vi "increasing temp.vi"() -> ()   [LabVIEW 2016]
panel:
  in  "X":cluster{"Y":dbl[], "Y":dbl[]}[](graph)=[{"Y"=[3642203376.678899, 3642203381.4529734, 3642203385.471007, 3642203389.0781093, 3642203393.010663, 3642203396.7724032, 3642203404.0189867, 3642203408.627992, 3642203413.007674, 3642203417.017978, 3642203421.7605133, 3642203425.9109974, 3642203430.7061076, 3642203434.9230328, 3642203438.9979987, 3642203443.332184, 3642203447.2605352, 3642203451.7941136, 3642203459.39853, 3642203467.88641, 3642203474.175996, 3642203481.486995, 3642203488.474578, 3642203496.3469887, 3642203503.9469843, 3642203511.239989, 3642203517.483984, 3642203524.005077, 3642203531.319994, 3642203537.588065, 3642203544.0179725, 3642203549.2159953, 3642203553.9432397, 3642203558.7595663, 3642203563.727993, 3642203568.8299923, 3642203574.1562724, 3642203579.535736, 3642203585.0829887, 3642203589.851984, 3642203595.764988, 3642203601.6856017, 3642203607.86395, 3642203614.0785565, 3642203620.498435, 3642203627.0719585, 3642203633.7784004, 3642203640.6264877, 3642203647.60899, 3642203654.7438607, 3642203662.021482, 3642203669.455943, 3642203676.9799685, 3642203684.697377, 3642203692.553962, 3642203700.53799, 3642203708.670955, 3642203716.9027405, 3642203725.309407, 3642203733.9799547, 3642203742.824001, 3642203750.447501, 3642203758.1655297, 3642203766.063456, 3642203774.020072, 3642203782.130978, 3642203790.362556, 3642203798.7464366, 3642203807.2065024, 3642203815.7734337, 3642203824.4805117, 3642203833.303608, 3642203840.6899595, 3642203849.7780876, 3642203858.9921017, 3642203868.3275275, 3642203877.7842393, 3642203887.371065, 3642203895.324416, 3642203905.134486, 3642203915.0885224, 3642203925.1429653, 3642203935.3679466, 3642203945.691629, 3642203956.1247206, 3642203966.6969767, 3642203977.389964, 3642203988.232658, 3642203999.2042, 3642204010.2849526, 3642204021.478747, 3642204032.8189797, 3642204044.2453103, 3642204055.819765, 3642204067.5106335, 3642204079.313611, 3642204091.2315116, 3642204103.2799654, 3642204115.4469485, 3642204127.6961465, 3642204140.073737, 3642204152.5979676, 3642204165.248852, 3642204178.006964, 3642204190.896954, 3642204203.954037, 3642204217.008529, 3642204230.282956, 3642204243.598564, 3642204257.1349783, 3642204270.7075243, 3642204284.50797, 3642204298.4340215, 3642204312.446953, 3642204326.5109596, 3642204340.7429686, 3642204355.0933547, 3642204369.543991, 3642204384.127608, 3642204398.8509536, 3642204413.676495, 3642204428.6227765, 3642204443.7505007, 3642204458.9438233, 3642204474.289527, 3642204489.754409, 3642204505.3876953, 3642204521.133424, 3642204536.981744, 3642204552.9799566], "Y"=[-4.592852846155305e-07, 6.737261391003903e-07, -1.6202429618948316e-07, -5.195699919208646e-07, 1.7745755993713474e-07, 3.0616714385976003e-08, -5.069567713584076e-07, -2.851272362169249e-06, 2.269853345124516e-07, -1.516212895524327e-07, 8.512614073389253e-07, -6.452557272346467e-08, -2.488638727511979e-08, -1.5909099540442844e-07, 2.141604585632381e-06, -5.713671338361288e-07, 1.838870943039606e-07, -6.85689824952017e-07, 4.4964985987086557e-07, 1.0277080054535237e-06, 1.8268333019083994e-06, 1.2651076458122845e-06, -1.9817887883287324e-06, 3.199258834789368e-06, -4.2675292042007555e-07, -3.157697760053565e-07, -1.8719773358338287e-07, 1.6720646447380741e-06, -2.105916273763826e-07, -2.148051334650441e-06, 2.371464662143136e-06, -2.2078978505204405e-07, 8.068317843909511e-07, 3.4287007154703245e-07, 3.3234889116131063e-06, 3.753292230747245e-07, -2.385901688203542e-06, 8.205820722248888e-07, -1.3887099455243955e-06, -9.231387346711631e-07, -3.913940073942008e-07, 7.028091024842494e-08, 4.1020767684091775e-07, 8.443503716354726e-08, 2.2321015092773138e-07, 7.953201420298254e-07, 1.1317495233520216e-07, 3.814309860176883e-07, 1.9994082382836704e-07, 9.937482494362683e-07, -1.8197887989598828e-07, 1.1392285669304173e-06, 6.804527296161199e-08, -1.6850208090832188e-06, -8.390044359649611e-08, -1.9510360617117507e-06, -3.7185186656709547e-07, 2.527165648808925e-06, -3.3413965856755106e-06, -3.872050452328565e-07, -2.4872526748053463e-08, -4.893893237121692e-07, -3.1804016518869365e-06, -1.4217086887640428e-06, 1.9969842700177657e-06, -2.03139815976751e-06, -2.783520563565814e-07, -5.461780301286425e-08, -3.6310779917499475e-06, 3.487828739949907e-08, 7.766851219627903e-07, -2.759841576063468e-06, 9.934826358592591e-07, -2.7691004013781596e-07, 8.031039004236865e-07, -5.728049833494833e-07, -8.426202455162954e-07, -8.950632140867222e-08, 3.306172369715688e-06, 1.2042888547753334e-06, -2.3981153221307364e-06, -3.688452875024709e-07, 2.5961297228656354e-07, -5.407344321405053e-07, -2.9150556743347184e-06, 3.653850715662323e-08, -9.539094741857481e-07, -1.3021341954056513e-06, 1.3108920889672774e-06, -4.906554468364315e-07, 2.403335962878498e-07, -3.7565399138340026e-08, -2.0821658466886e-07, -6.784523874482342e-07, -2.5919522452637248e-06, 2.1004599285403896e-06, -2.2889086103393647e-08, -2.1428098028062635e-07, -2.423515211069741e-07, -1.7162037979416079e-06, 9.163286643010077e-07, -4.369004096472446e-07, -1.4447923111259159e-08, -2.5202656790406694e-06, 8.073623013821671e-07, 1.8036487500392036e-06, 1.0001897464779398e-07, 1.129728924637367e-06, 8.361201946413808e-07, 2.383023409974057e-06, 3.589627808873978e-07, -1.9274590125012865e-06, 8.983752650375939e-07, -2.9701301720357084e-07, -4.421372824968631e-08, 2.993917059194213e-07, -1.739131561173571e-08, -2.479915285148134e-06, 5.942825402414524e-07, -2.1677077419945556e-06, -1.0154454404227488e-06, -4.293038866311916e-07, 2.1474063832532374e-06, -2.6065890098976974e-07, -1.7457701197748126e-07, -2.8440312787674336e-07, -1.5603054734035735e-06, -7.222947430545974e-07, -5.038970456553111e-08, 5.216494419849221e-07]}, ...(8 in all)]
  in  "R vs time":cluster{"Y":dbl[], "Y":dbl[]}[](graph)=[{"Y"=[3642203376.678899, 3642203381.4529734, 3642203385.471007, 3642203389.0781093, 3642203393.010663, 3642203396.7724032, 3642203404.0189867, 3642203408.627992, 3642203413.007674, 3642203417.017978, 3642203421.7605133, 3642203425.9109974, 3642203430.7061076, 3642203434.9230328, 3642203438.9979987, 3642203443.332184, 3642203447.2605352, 3642203451.7941136, 3642203459.39853, 3642203467.88641, 3642203474.175996, 3642203481.486995, 3642203488.474578, 3642203496.3469887, 3642203503.9469843, 3642203511.239989, 3642203517.483984, 3642203524.005077, 3642203531.319994, 3642203537.588065, 3642203544.0179725, 3642203549.2159953, 3642203553.9432397, 3642203558.7595663, 3642203563.727993, 3642203568.8299923, 3642203574.1562724, 3642203579.535736, 3642203585.0829887, 3642203589.851984, 3642203595.764988, 3642203601.6856017, 3642203607.86395, 3642203614.0785565, 3642203620.498435, 3642203627.0719585, 3642203633.7784004, 3642203640.6264877, 3642203647.60899, 3642203654.7438607, 3642203662.021482, 3642203669.455943, 3642203676.9799685, 3642203684.697377, 3642203692.553962, 3642203700.53799, 3642203708.670955, 3642203716.9027405, 3642203725.309407, 3642203733.9799547, 3642203742.824001, 3642203750.447501, 3642203758.1655297, 3642203766.063456, 3642203774.020072, 3642203782.130978, 3642203790.362556, 3642203798.7464366, 3642203807.2065024, 3642203815.7734337, 3642203824.4805117, 3642203833.303608, 3642203840.6899595, 3642203849.7780876, 3642203858.9921017, 3642203868.3275275, 3642203877.7842393, 3642203887.371065, 3642203895.324416, 3642203905.134486, 3642203915.0885224, 3642203925.1429653, 3642203935.3679466, 3642203945.691629, 3642203956.1247206, 3642203966.6969767, 3642203977.389964, 3642203988.232658, 3642203999.2042, 3642204010.2849526, 3642204021.478747, 3642204032.8189797, 3642204044.2453103, 3642204055.819765, 3642204067.5106335, 3642204079.313611, 3642204091.2315116, 3642204103.2799654, 3642204115.4469485, 3642204127.6961465, 3642204140.073737, 3642204152.5979676, 3642204165.248852, 3642204178.006964, 3642204190.896954, 3642204203.954037, 3642204217.008529, 3642204230.282956, 3642204243.598564, 3642204257.1349783, 3642204270.7075243, 3642204284.50797, 3642204298.4340215, 3642204312.446953, 3642204326.5109596, 3642204340.7429686, 3642204355.0933547, 3642204369.543991, 3642204384.127608, 3642204398.8509536, 3642204413.676495, 3642204428.6227765, 3642204443.7505007, 3642204458.9438233, 3642204474.289527, 3642204489.754409, 3642204505.3876953, 3642204521.133424, 3642204536.981744, 3642204552.9799566], "Y"=[-13290.384994182137, 1010.1645943186124, 230.8834081303573, 505.0614514743513, -455.87875652676956, -347.65742757917116, -198.8157632722718, 115.53565091546876, 69.86024909637129, 685.9043843352671, 127.54203131523417, -265.0436708966293, 1027.8647107628037, 98.26066311690617, -90.35268828461413, -376.2284141948499, 88.03611307741558, -145.34812417196756, -1553.3499581145566, 326.96215862747954, -438.83393132227064, 314.48409646060975, -227.89771600863875, -285.20090012475526, -225.7743279866675, 894.151046847666, 85.48750599653887, 94.19871267267854, -3151.030530979217, -183.8518031082741, 107.75310480616433, -308.7289092302942, -76.9274657912896, 506.7721395612492, 154.73306778906723, -279.1402317310842, 68.65915413987439, 78.47527046278749, -233.22981679751558, 136.24621089711266, -463.73522280732885, 918.4952239414861, 124.17496153076863, 1757.6820722657455, -99.39510800194688, 474.16223699786786, -5607.487297384516, 3384.8904626708536, -137.41017892314042, 106.14751920160279, 328.9636349711561, 69.88530464928033, -274.31526774598325, 421.52639724158934, -270.7268804214494, 111.31495180204152, 64.12456724666644, -133.11753372504052, 111.75367259286068, -115.32654979456255, 677.85032755026, -225.8089492085577, 382.76642181163135, 65.25075622172892, 149.52420762427815, -141.94191274768636, 793.6913983817947, 165.48311983637146, 107.88964964815528, -274.1442371616069, 266.9324173776331, -250.10815522287393, 451.8262632447018, 367.75400371050847, 358.2816983530076, 143.47953484189077, 377.59372738687733, -186.41234302891658, 646.5059539950425, 339.06642810760894, -189.9145337439248, -191.8504902624153, -92.5078518800701, 116.53997824125695, 782.0683466334028, 83.4544598367022, 46.62644153088291, -139.67077157215348, 79.06391418478647, -85.01404321215314, 635.5607371774844, -167.36909150226882, 124.9096566032149, -988.8938244735011, -84.45157127001838, -285.99359282222133, -277.7605421719423, 174.17733462504447, 75.31875398945978, 108.37819654495885, -495.0486671057887, -86.2722362352597, 99.91213152958176, -775.2594739404896, -118.77363531096636, -101.02457531539693, -37074.070699578064, -88.40258250374514, -289.58175041371396, 70.09699762089551, -132.2993403840001, -71.21000706288028, 144.4705388929231, 82.59029107319097, 98.64970050315146, -99.91347933530021, -796.6980670694059, 3741.1270720067746, -86.07941304594911, 63.43702018971397, -107.47009692561538, 646.3220418964175, -144.94610473502064, 110.80438801802686, 146.3562135553641, 84.5214660465581, 708.4113116150547, -125.80004750025807, -111.36372341699885, -167.778772663313]}, {"Y"=[3642203376.678899, 3642203381.4529734, 3642203385.471007, 3642203389.0781093, 3642203393.010663, 3642203396.7724032, 3642203404.0189867, 3642203408.627992, 3642203413.007674, 3642203417.017978, 3642203421.7605133, 3642203425.9109974, 3642203430.7061076, 3642203434.9230328, 3642203438.9979987, 3642203443.332184, 3642203447.2605352, 3642203451.7941136, 3642203459.39853, 3642203467.88641, 3642203474.175996, 3642203481.486995, 3642203488.474578, 3642203496.3469887, 3642203503.9469843, 3642203511.239989, 3642203517.483984, 3642203524.005077, 3642203531.319994, 3642203537.588065, 3642203544.0179725, 3642203549.2159953, 3642203553.9432397, 3642203558.7595663, 3642203563.727993, 3642203568.8299923, 3642203574.1562724, 3642203579.535736, 3642203585.0829887, 3642203589.851984, 3642203595.764988, 3642203601.6856017, 3642203607.86395, 3642203614.0785565, 3642203620.498435, 3642203627.0719585, 3642203633.7784004, 3642203640.6264877, 3642203647.60899, 3642203654.7438607, 3642203662.021482, 3642203669.455943, 3642203676.9799685, 3642203684.697377, 3642203692.553962, 3642203700.53799, 3642203708.670955, 3642203716.9027405, 3642203725.309407, 3642203733.9799547, 3642203742.824001, 3642203750.447501, 3642203758.1655297, 3642203766.063456, 3642203774.020072, 3642203782.130978, 3642203790.362556, 3642203798.7464366, 3642203807.2065024, 3642203815.7734337, 3642203824.4805117, 3642203833.303608, 3642203840.6899595, 3642203849.7780876, 3642203858.9921017, 3642203868.3275275, 3642203877.7842393, 3642203887.371065, 3642203895.324416, 3642203905.134486, 3642203915.0885224, 3642203925.1429653, 3642203935.3679466, 3642203945.691629, 3642203956.1247206, 3642203966.6969767, 3642203977.389964, 3642203988.232658, 3642203999.2042, 3642204010.2849526, 3642204021.478747, 3642204032.8189797, 3642204044.2453103, 3642204055.819765, 3642204067.5106335, 3642204079.313611, 3642204091.2315116, 3642204103.2799654, 3642204115.4469485, 3642204127.6961465, 3642204140.073737, 3642204152.5979676, 3642204165.248852, 3642204178.006964, 3642204190.896954, 3642204203.954037, 3642204217.008529, 3642204230.282956, 3642204243.598564, 3642204257.1349783, 3642204270.7075243, 3642204284.50797, 3642204298.4340215, 3642204312.446953, 3642204326.5109596, 3642204340.7429686, 3642204355.0933547, 3642204369.543991, 3642204384.127608, 3642204398.8509536, 3642204413.676495, 3642204428.6227765, 3642204443.7505007, 3642204458.9438233, 3642204474.289527, 3642204489.754409, 3642204505.3876953, 3642204521.133424, 3642204536.981744, 3642204552.9799566], "Y"=[-132796.6116027698, 10085.227856625914, 2307.0294179465814, 5039.729604322662, -4554.452571861353, -3472.086936251539, -1985.381474922613, 1152.3611036806205, 696.300133797407, 6841.098888724538, 1273.2972821711066, -2649.792976557507, 10263.659053433017, 980.0204104096836, -905.7400995754302, -3764.276215915255, 877.6946943017681, -1454.7366170262428, -15508.540436514326, 3264.539414175311, -4386.274426303269, 3138.3216518011777, -2283.471602003312, -2857.714376475587, -2266.9573832255073, 8923.190205933595, 848.8811251358674, 934.196123590157, -31692.60099539315, -1850.80455337936, 1070.8179155334785, -3088.601183974256, -774.3799299013517, 5063.068159695625, 1541.6634936536605, -2801.5948108459747, 679.2769340091177, 775.1587147638663, -2340.2446211602314, 1356.8419370937438, -4658.911887974246, 9159.128327924667, 1233.9862130578044, 17540.558227007925, -1000.2367117690112, 4713.895693647603, -55888.02334250651, 33684.91158899502, -1378.8104866306774, 1055.5447747562584, 3278.5822649935185, 695.0494692381241, -2734.069788924536, 4223.884439343381, -2706.9796851271935, 1108.3484042355785, 636.0306546233915, -1334.3117017862949, 1110.6279797090228, -1157.816758776485, 6774.944907780769, -2255.0989351931994, 3812.9040611672635, 648.1933415744867, 1490.7479408990548, -1421.7872356767666, 7927.3269304686955, 1648.817290193451, 1073.0456327825368, -2744.479414586225, 2666.1936399496394, -2504.0793939382265, 4503.890730740483, 3673.3393501643573, 3584.0012889508434, 1428.891725304976, 3767.419431889385, -1866.3263080023928, 6440.03489668795, 3385.7200750420943, -1901.7673363744577, -1920.0878596017894, -927.3684535328207, 1160.4379123000112, 7805.78117474216, 829.7770089001393, 463.71411717091223, -1398.514952017124, 787.3738262761995, -852.5225233200302, 6337.868651185304, -1676.6891609434108, 1245.588796869341, -9878.588491395047, -848.0576467816252, -2865.340182192463, -2774.7489127649087, 1735.9454896524096, 749.9226021314499, 1078.8685051502137, -4954.1708846236925, -865.3622872178395, 994.1359126982633, -7744.246036537609, -1188.3752639042932, -1011.6358138074454, -371442.7147593308, -887.0372385422618, -2899.0577725548264, 696.1003393609519, -1327.9696437364057, -716.3856883124266, 1436.570653460954, 821.7308491830619, 980.0240580012867, -1003.1834429756749, -7971.8512521816765, 37418.84161607035, -865.7351880955226, 627.6636246451059, -1077.13661963261, 6429.216978225116, -1457.5368446306697, 1100.0766225267735, 1455.0156258309783, 838.8898084608107, 7065.980965670538, -1262.1693495487746, -1119.1475300528555, -1682.0807347958]}]
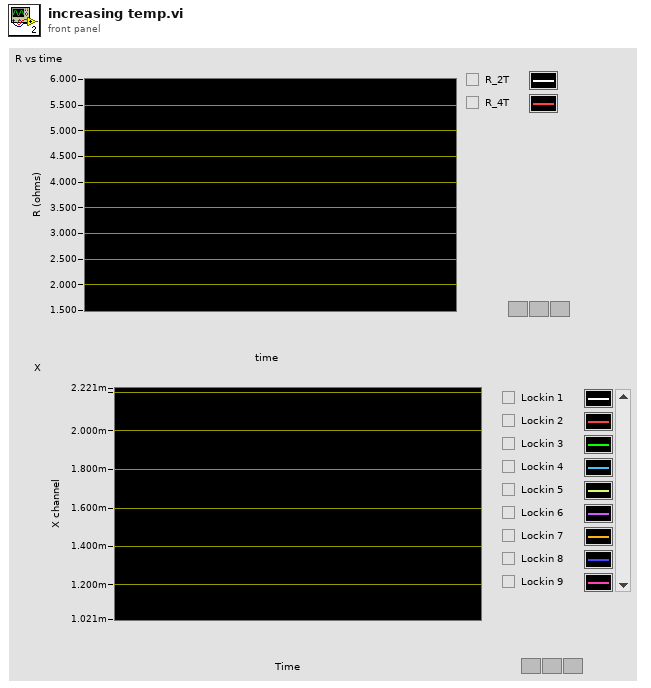
[diagram p1: front panel]
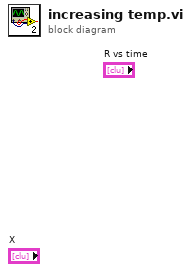
[diagram p0: block diagram]
diagram:
